vi "Frisbee Counter.vi"   [LabVIEW 2012]
uses:
  BotStatus.vi
types:
  T1 = cluster{"Middle":bool, "InFlipper":bool, "Bottom":bool, "FlipperDown":bool, "Frizbee Counter":dbl}
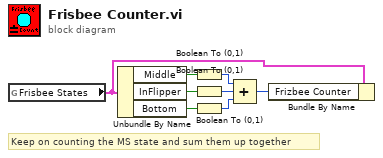
[diagram p0: block diagram]
diagram:
  # "Keep on counting the MS state and sum them up together"
  n1 = global read "BotStatus.vi" "Frisbee States"() -> (w8:T1)
  n2 = Unbundle By Name(w8) -> ("Middle"=w1:bool, "InFlipper"=w2:bool, "Bottom"=w3:bool)
  n3 = Boolean To (0,1)(Boolean=w1) -> (0, 1=w4:i16)
  n4 = Boolean To (0,1)(Boolean=w2) -> (0, 1=w6:i16)
  n5 = Boolean To (0,1)(Boolean=w3) -> (0, 1=w5:i16)
  n6 = Compound Arithmetic op=ADD(w4, w6, w5) -> (w7:i16)
  n7 = Bundle By Name(cluster=w8, "Frizbee Counter"=w7) -> ()  [unwired: 1 out]
